vi "Verify Mock.vi"(8 "error in (no error)":errorcluster, 11 "Mock In":refnum<class "LMock Mock.lvclass">) -> (0 "error out":errorcluster, 1 "Errors":errorcluster[](array[cluster]), 2 "Results":cluster{"Passed?":bool, "Message":string}[](array[cluster]))   [LabVIEW 2020, in "LMock Mock.lvclass"]
uses:
  LMock Mock.lvclass
  LMock Mock.lvclass/LMock Mock.ctl
  Core/Expectation/Expectation.lvclass
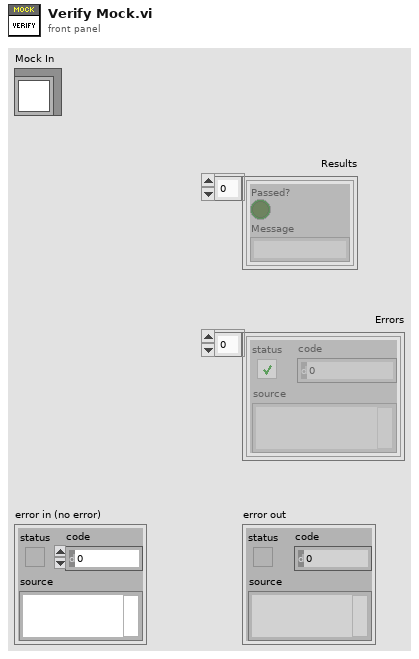
[diagram p1: front panel]
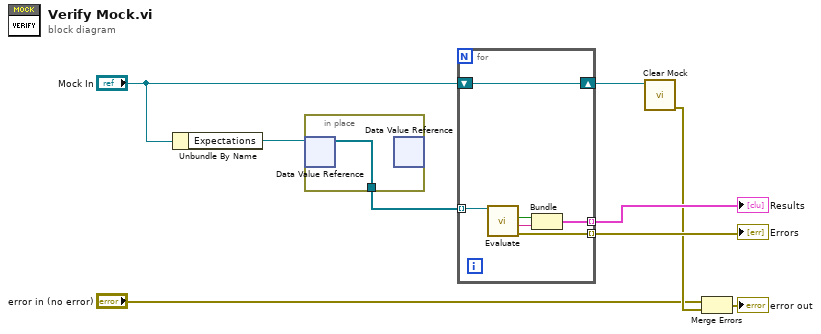
[diagram p0: block diagram]
diagram:
  n1 = Unbundle By Name("Mock In") -> ("Expectations"=w6:refnum<data-value>)
  n2 = in-place {
    in-place-border: [w10] -> w7
    n3 = in-place-dvr #1(w6) -> (w10:refnum<class "Expectation.lvclass">[])  [unwired: 1 out]
    n4 = in-place-dvr #1() -> ()  [unwired: 1 in, 2 out]
  }
  n5 = for {
    tunnel: [w16] -> w9 mode=indexing
    tunnel: w7 -> [w15] mode=indexing
    tunnel: [w12] -> w8 mode=indexing
    shift-right: [w11] -> w1
    shift-left: "Mock In" -> [w11]
    n6 = call-dynamic "Evaluate.vi"("Expectation in"=w15) -> ("error out"=w16:errorcluster, "Message"=w13:string, "Passed?"=w14:bool)  [unwired: 8 in]
    n7 = Bundle("Passed?"=w14, "Message"=w13) -> (w12:cluster{"Passed?":bool, "Message":string})  [unwired: 1 in]
  }
  "Errors" <- w9
  "Results" <- w8
  n8 = call-dynamic "Clear Mock.vi"("Mock In"=w1) -> ("error out"=w5:errorcluster)  [unwired: 10 in]
  n9 = Merge Errors("error in (no error)", w5) -> (→"error out":errorcluster)
